vi "Write ElectrometerConfiguration.vi"(8 "error in (no error)":errorcluster, 10 "ElectrometerConfiguration":refnum<class "ElectrometerCOMConfiguration.lvclass">, 11 "Electrometer in":refnum<class "Electrometer.lvclass">) -> (0 "error out":errorcluster, 3 "Electrometer out":refnum<class "Electrometer.lvclass">)   [LabVIEW 2016, in "Electrometer.lvclass"]
uses:
  Electrometer.lvclass
  ElectrometerConfiguration/ElectrometerCOMConfiguration.lvclass
  Electrometer.lvclass/Electrometer.ctl
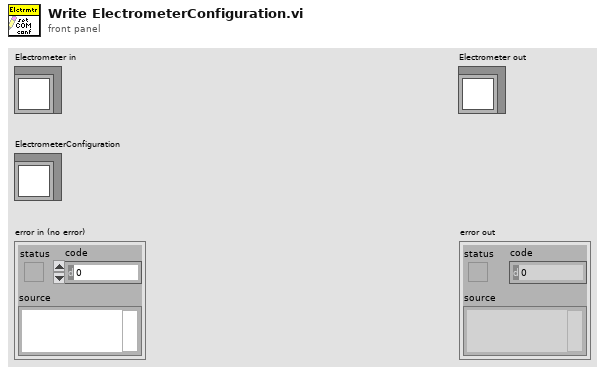
[diagram p1: front panel]
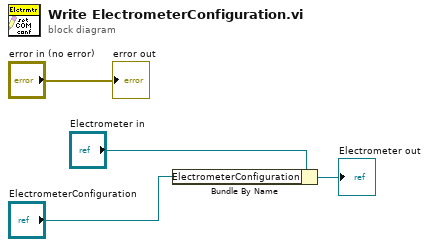
[diagram p0: block diagram]
diagram:
  n1 = Bundle By Name(cluster="Electrometer in", "ElectrometerConfiguration"="ElectrometerConfiguration") -> (→"Electrometer out":refnum<class "Electrometer.lvclass">)
  "error out" <- "error in (no error)"
